vi "getRunPath.vi"(8 "error in (no error)":errorcluster, 11 "StaticOutputEditor in":refnum<class "StaticOutputEditor.lvclass">) -> (0 "error out":errorcluster, 1 "runParameter":string, 2 "Path":path, 3 "StaticOutputEditor out":refnum<class "StaticOutputEditor.lvclass">)   [LabVIEW 2009, in "Views.lvlib" / "ScriptEditor.lvlib" / "StaticOutputEditor.lvclass"]
uses:
  StaticOutputEditor.lvclass
  Tools/Filing/FileSystem/FileSystem.lvclass
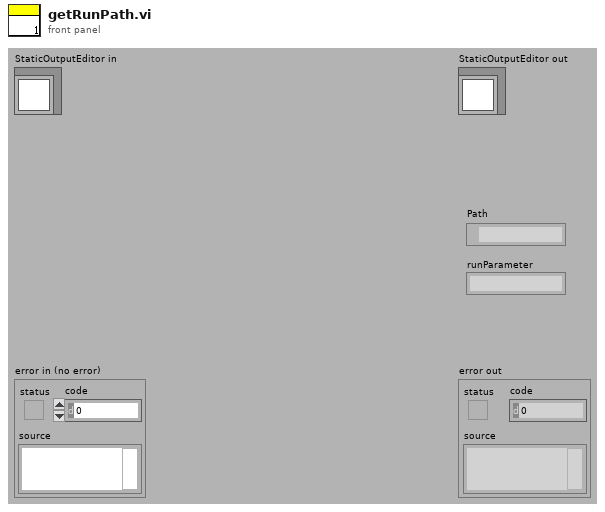
[diagram p1: front panel]
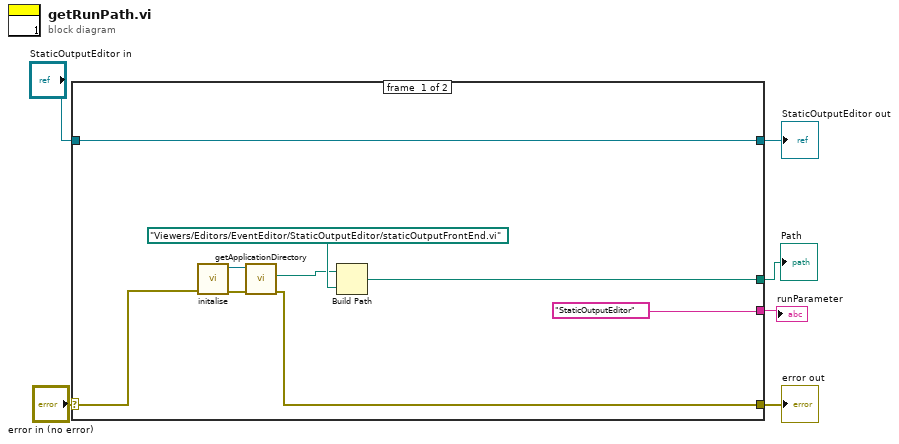
[diagram p0: block diagram]
diagram:
  n1 = case shown="No Error" "error in (no error)" {
    selector: "error in (no error)" -> [w9 w17]
    tunnel: [w8 w17] -> w5
    tunnel: [w15 w16] -> w3
    tunnel: "StaticOutputEditor in" -> [w15 w16]
    tunnel: [w10 _] -> w2
    tunnel: ["StaticOutputEditor" _] -> w1
    frame #0 {
      n2 = call "initalise.vi"("error in (no error)"=w9) -> ("error out"=w13:errorcluster, "FileSystem out"=w14:refnum<class "FileSystem.lvclass">)  [unwired: 9 in]
      n3 = call-dynamic "getApplicationDirectory.vi"("error in (no error)"=w13, "FileSystem.lvclass in"=w14) -> ("error out"=w8:errorcluster, "ApplicationDirectory"=w11:path)  [unwired: 7 in, 1 out]
      n4 = Build Path(base path=w11, name or relative path=path "Viewers/Editors/EventEditor/StaticOutputEditor/staticOutputFrontEnd.vi" ("vi path")) -> (appended path=w10:path)
    }
    frame #1 {
    }
  }
  "error out" <- w5
  "StaticOutputEditor out" <- w3
  "Path" <- w2
  "runParameter" <- w1
